vi "Read Spec Page Path.vi"(8 "error in":errorcluster, 11 "NIVS_CDEW_MetaDataObj in":refnum<class "NIVS_CDEW_MetaDataObj.lvclass">) -> (0 "error out":errorcluster, 2 "Spec Page VI Path":path, 3 "NIVS_CDEW_MetaDataObj out":refnum<class "NIVS_CDEW_MetaDataObj.lvclass">)   [LabVIEW 2026, in "NIVS_CDEW_MetaDataObj.lvclass"]
uses:
  NIVS_CDEW_MetaDataObj.lvclass
  NIVS_CDEW_MetaDataObj.lvclass/NIVS_CDEW_MetaDataObj.ctl
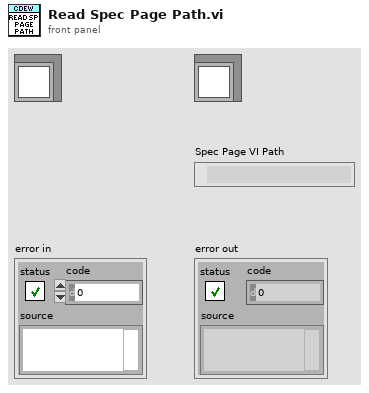
[diagram p1: front panel]
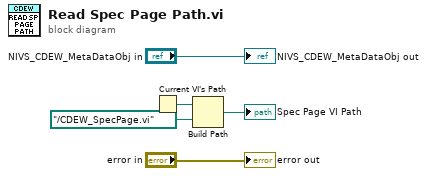
[diagram p0: block diagram]
diagram:
  n1 = Current VI's Path() -> (path=w3:path)
  n2 = Build Path(base path=w3, name or relative path=path "../CDEW_SpecPage.vi") -> (appended path=→"Spec Page VI Path":path)
  "error out" <- "error in"
  "NIVS_CDEW_MetaDataObj out" <- "NIVS_CDEW_MetaDataObj in"
